vi "driveToCreateCommands.vi"(6 "toGuidedDrive":bool, 8 "toFreestyle":bool, 9 "toDriveDistance":bool, 10 "toTurnAngle":bool, 11 "toReserve":bool) -> (3 "Current State":T1)   [LabVIEW 2017]
uses:
  Implementation/Drive Operations.ctl
  <vilib>/FRCT Team# 3937  Breakaway/Memory Library/memLib.lvlib
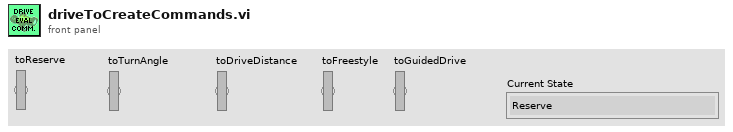
[diagram p1: front panel]
types:
  T1 = typedef "Drive Operations.ctl" = enum16{"Reserve", "Read Current", "Freestyle", "Drive for Distance", "TurnAngle", "Guided Drive"}
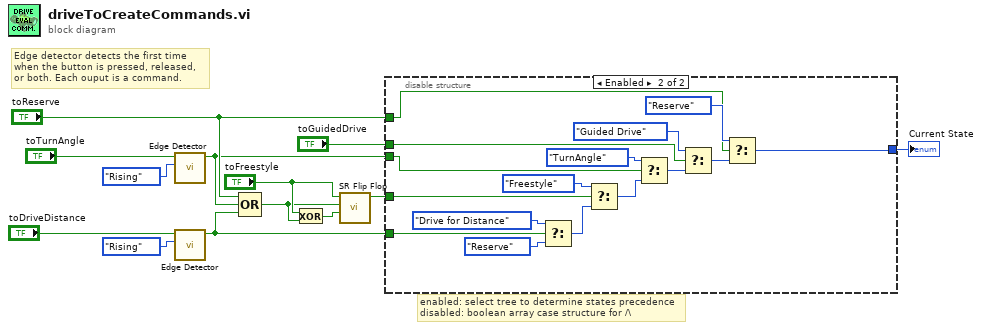
[diagram p0: block diagram]
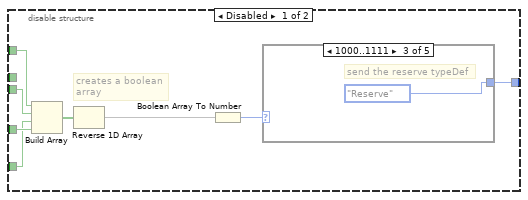
[diagram p2: hidden frame]
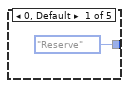
[diagram p3: hidden frame]
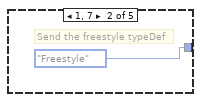
[diagram p4: hidden frame]
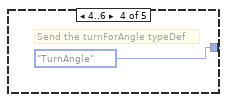
[diagram p5: hidden frame]
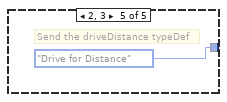
[diagram p6: hidden frame]
diagram:
  # "enabled: select tree to determine states precedence\ndisabled: boolean array case structure for /\\"
  # "Edge detector detects the first time\nwhen the button is pressed, released,\nor both. Each ouput is a command."
  n1 = call <vilib>:"Edge Detector.vi"("Mode"=enum16{"Rising", "Falling", "Any"}."Rising", "Input"="toTurnAngle") -> ("Output"=w8:bool)  [unwired: 9 in]
  n2 = call <vilib>:"Edge Detector.vi"("Mode"=enum16{"Rising", "Falling", "Any"}."Rising", "Input"="toDriveDistance") -> ("Output"=w3:bool)  [unwired: 9 in]
  n3 = Compound Arithmetic op=OR("toReserve", w8, w3) -> (w6:bool)
  n4 = Exclusive Or(1:w6, 2:"toFreestyle") -> (0:w5:bool)
  n5 = call <vilib>:"SR Flip Flop.vi"("Enable"=w5, "Reset"=w6, "Set"="toFreestyle") -> ("Output"=w10:bool)  [unwired: 8 in]
  n6 = disable-structure shown="Enabled" {
    disable-tunnel: w10 -> [w18 w34]
    disable-tunnel: "toReserve" -> [w17 w35]
    disable-tunnel: w8 -> [w16 w33]
    disable-tunnel: w3 -> [w15 w32]
    disable-tunnel: [w14 w41] -> w2
    disable-tunnel: "toGuidedDrive" -> [_ w31]
    frame Disabled {
      # "creates a boolean\narray"
      n7 = Build Array(w17, w16, w15, w18) -> (w20:bool[])
      n8 = Reverse 1D Array(array=w20) -> (reversed array=w19:bool[])
      n9 = Boolean Array To Number(Boolean array=w19) -> (number=w21:u32)
      n10 = case shown="1000..1111" w21 {
        tunnel: [Drive_Operations."Reserve" ("Enum") Drive_Operations."Freestyle" ("Enum") Drive_Operations."Reserve" ("Enum") Drive_Operations."TurnAngle" ("Enum") Drive_Operations."Drive for Distance" ("Enum")] -> w14
        frame 0, Default {
        }
        frame 1, 7 {
          # "Send the freestyle typeDef"
        }
        frame 8..15 {
          # "send the reserve typeDef"
        }
        frame 4..6 {
          # "Send the turnForAngle typeDef"
        }
        frame 2, 3 {
          # "Send the driveDistance typeDef"
        }
      }
    }
    frame Enabled {
      n11 = Select(t=Drive_Operations."Drive for Distance" ("Enum"), s=w32, f=Drive_Operations."Reserve" ("Enum")) -> (s? t:f=w28:T1)
      n12 = Select(t=Drive_Operations."Freestyle" ("Enum"), s=w34, f=w28) -> (s? t:f=w27:T1)
      n13 = Select(t=Drive_Operations."TurnAngle" ("Enum"), s=w33, f=w27) -> (s? t:f=w29:T1)
      n14 = Select(t=Drive_Operations."Guided Drive" ("Enum"), s=w31, f=w29) -> (s? t:f=w30:T1)
      n15 = Select(t=Drive_Operations."Reserve" ("Enum"), s=w35, f=w30) -> (s? t:f=w41:T1)
    }
  }
  "Current State" <- w2
